vi "recipeScript getScriptInfo.vi"(0 "sysCode":string, 1 "method":T1) -> (3 "output":string)   [LabVIEW 2018]
uses:
  getScriptInfo.ctl
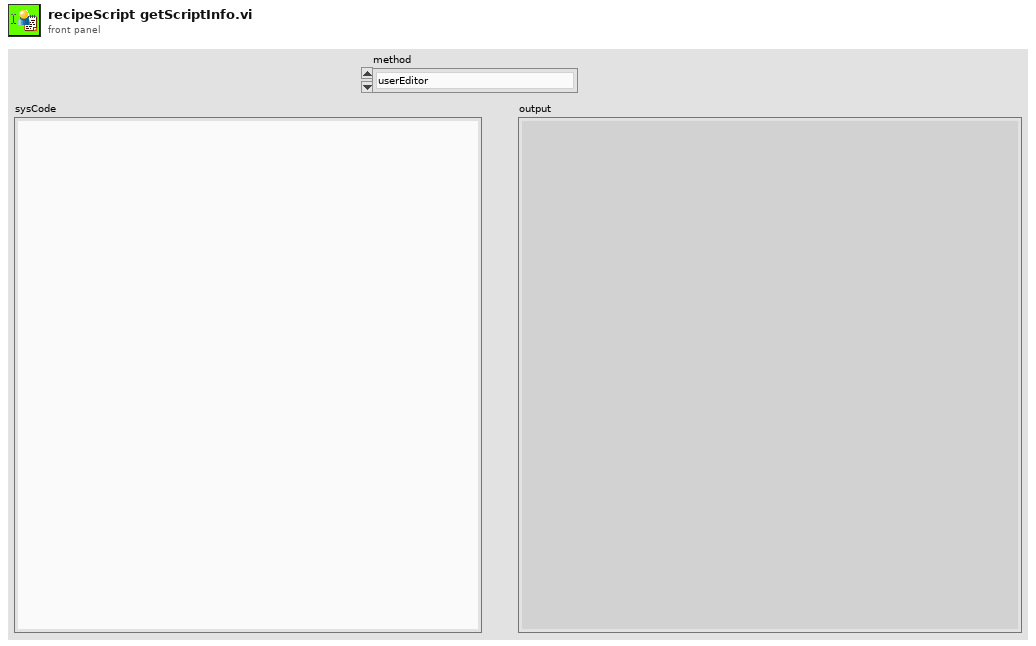
[diagram p1: front panel]
types:
  T1 = typedef "getScriptInfo.ctl" = enum16{"userEditor", "userParam", "instrParam", "sourcePath", "sourceTimeStamp", "versionInfo"}
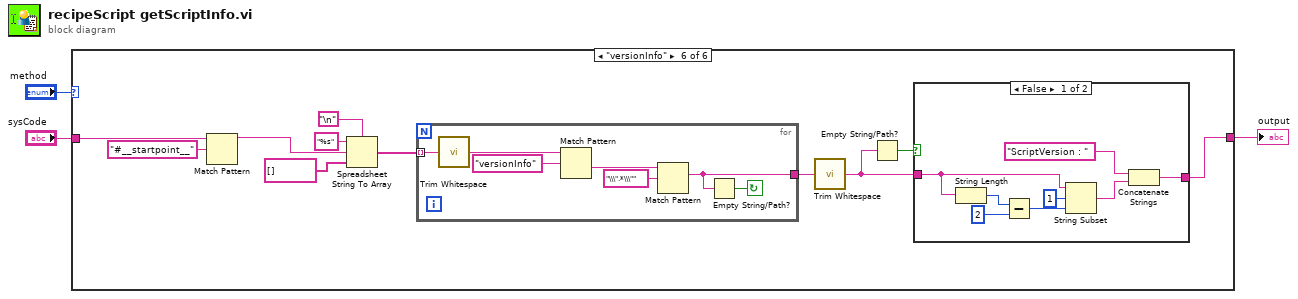
[diagram p0: block diagram]
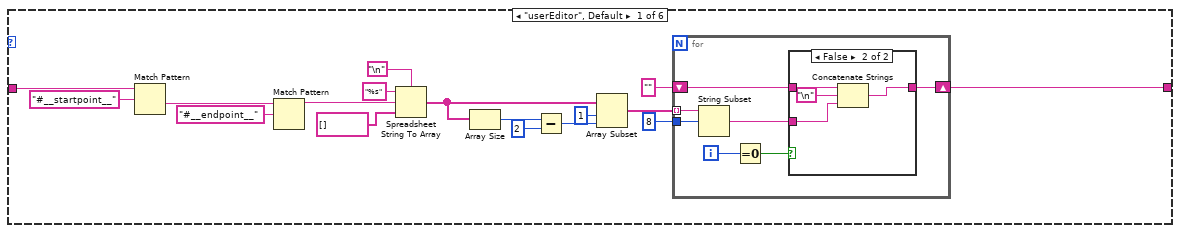
[diagram p2: hidden frame]
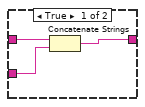
[diagram p3: hidden frame]
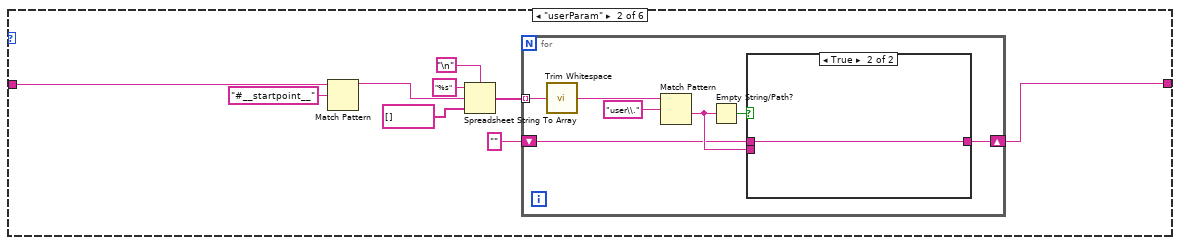
[diagram p4: hidden frame]
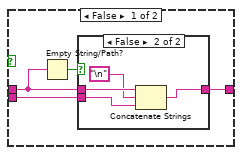
[diagram p5: hidden frame]
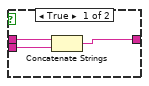
[diagram p6: hidden frame]
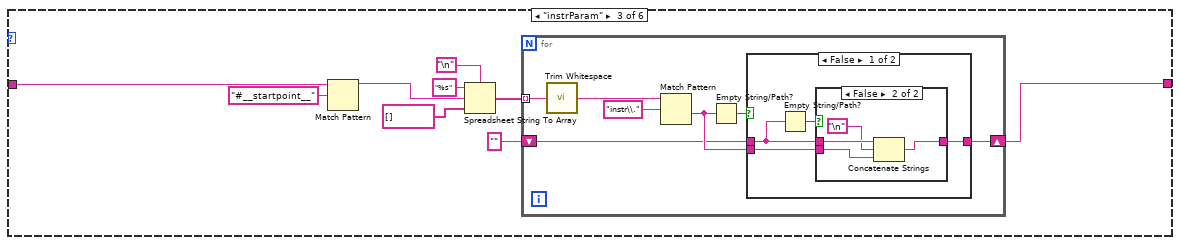
[diagram p7: hidden frame]
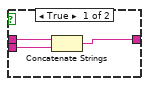
[diagram p8: hidden frame]
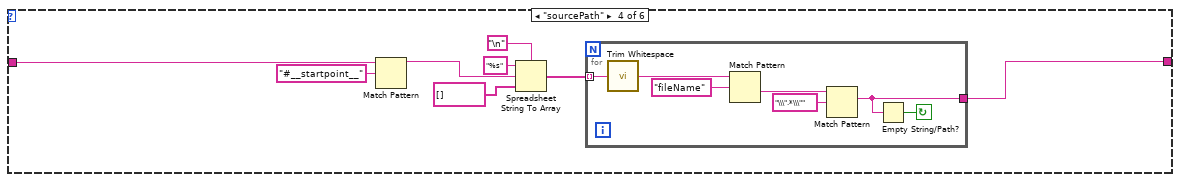
[diagram p10: hidden frame]
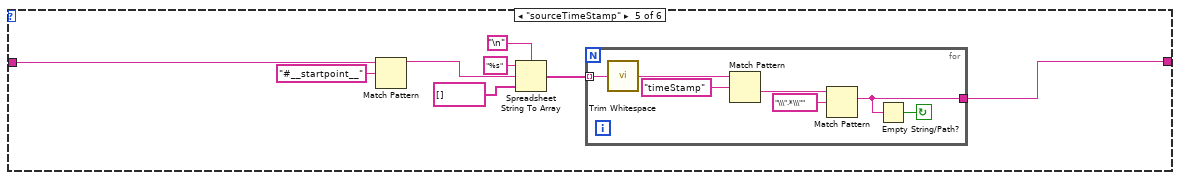
[diagram p11: hidden frame]
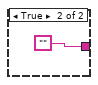
[diagram p12: hidden frame]
diagram:
  n1 = case shown="\"versionInfo\"" "method" {
    tunnel: "sysCode" -> [w20 w35 w63 w91 w106 w125]
    tunnel: [w8 w36 w64 w92 w107 w121] -> w2
    frame "userEditor", Default {
      n2 = Match Pattern(string=w20, regular expression="#__startpoint__") -> (after substring=w7:string)  [unwired: 1 in, 3 out]
      n3 = Match Pattern(string=w7, regular expression="#__endpoint__") -> (before substring=w5:string)  [unwired: 1 in, 3 out]
      n4 = Spreadsheet String To Array(delimiter (Tab)="\n", format string="%s", spreadsheet string=w5, array type (2D Dbl)=string[] []) -> (array=w14:string[])
      n5 = Array Size(array=w14) -> (size(s)=w13:i32)
      n6 = Subtract(x=w13, y=2) -> (x-y=w11:i32)
      n7 = Array Subset(array=w14, index=1, length=w11) -> (w10:string[])
      n8 = for {
        tunnel: w10 -> [w23] mode=indexing
        shift-right: [w26] -> w8
        shift-left: "" -> [w27]
        tunnel: 8 ("offset (0)") -> [w22]
        i -> [w25]
        n9 = String Subset(string=w23, offset (0)=w22) -> (substring=w21:string)  [unwired: 1 in]
        n10 = Equal To 0?(x=w25) -> (x = 0?=w24:bool)
        n11 = case shown="False" w24 {
          tunnel: w27 -> [w30 w34]
          tunnel: [w29 w33] -> w26
          tunnel: w21 -> [w28 w32]
          frame True {
            n12 = Concatenate Strings(w30, w28) -> (w29:string)
          }
          frame False {
            n13 = Concatenate Strings(w34, "\n", w32) -> (w33:string)
          }
        }
      }
    }
    frame "userParam" {
      n14 = Match Pattern(string=w35, regular expression="#__startpoint__") -> (before substring=w39:string)  [unwired: 1 in, 3 out]
      n15 = Spreadsheet String To Array(delimiter (Tab)="\n", format string="%s", spreadsheet string=w39, array type (2D Dbl)=string[] []) -> (array=w38:string[])
      n16 = for {
        tunnel: w38 -> [w50] mode=indexing
        shift-right: [w45] -> w36
        shift-left: "" -> [w44]
        n17 = call <vilib>:"Trim Whitespace.vi"("string"=w50) -> ("trimmed string"=w49:string)  [unwired: 1 in]
        n18 = Match Pattern(string=w49, regular expression="user\\.") -> (after substring=w46:string)  [unwired: 1 in, 3 out]
        n19 = Empty String/Path?(string/path=w46) -> (empty?=w47:bool)
        n20 = case shown="True" w47 {
          tunnel: w44 -> [w52 w62]
          tunnel: w46 -> [w54 _]
          tunnel: [w53 w62] -> w45
          frame False {
            n21 = Empty String/Path?(string/path=w52) -> (empty?=w51:bool)
            n22 = case shown="False" w51 {
              tunnel: w52 -> [w57 w61]
              tunnel: w54 -> [w56 w58]
              tunnel: [w55 w60] -> w53
              frame True {
                n23 = Concatenate Strings(w57, w56) -> (w55:string)
              }
              frame False {
                n24 = Concatenate Strings(w61, "\n", w58) -> (w60:string)
              }
            }
          }
          frame True {
          }
        }
      }
    }
    frame "instrParam" {
      n25 = Match Pattern(string=w63, regular expression="#__startpoint__") -> (before substring=w67:string)  [unwired: 1 in, 3 out]
      n26 = Spreadsheet String To Array(delimiter (Tab)="\n", format string="%s", spreadsheet string=w67, array type (2D Dbl)=string[] []) -> (array=w66:string[])
      n27 = for {
        tunnel: w66 -> [w78] mode=indexing
        shift-right: [w73] -> w64
        shift-left: "" -> [w72]
        n28 = call <vilib>:"Trim Whitespace.vi"("string"=w78) -> ("trimmed string"=w77:string)  [unwired: 1 in]
        n29 = Match Pattern(string=w77, regular expression="instr\\.") -> (after substring=w74:string)  [unwired: 1 in, 3 out]
        n30 = Empty String/Path?(string/path=w74) -> (empty?=w75:bool)
        n31 = case shown="False" w75 {
          tunnel: w72 -> [w80 w90]
          tunnel: w74 -> [w82 _]
          tunnel: [w81 w90] -> w73
          frame False {
            n32 = Empty String/Path?(string/path=w80) -> (empty?=w79:bool)
            n33 = case shown="False" w79 {
              tunnel: w80 -> [w85 w89]
              tunnel: w82 -> [w84 w86]
              tunnel: [w83 w88] -> w81
              frame True {
                n34 = Concatenate Strings(w85, w84) -> (w83:string)
              }
              frame False {
                n35 = Concatenate Strings(w89, "\n", w86) -> (w88:string)
              }
            }
          }
          frame True {
          }
        }
      }
    }
    frame "sourcePath" {
      n36 = Match Pattern(string=w91, regular expression="#__startpoint__") -> (before substring=w94:string)  [unwired: 1 in, 3 out]
      n37 = Spreadsheet String To Array(delimiter (Tab)="\n", format string="%s", spreadsheet string=w94, array type (2D Dbl)=string[] []) -> (array=w93:string[])
      n38 = for {
        tunnel: w93 -> [w103] mode=indexing
        tunnel: [w100] -> w92
        stop <- w99 continue-if-true
        n39 = call <vilib>:"Trim Whitespace.vi"("string"=w103) -> ("trimmed string"=w105:string)  [unwired: 1 in]
        n40 = Match Pattern(string=w105, regular expression="fileName") -> (after substring=w102:string)  [unwired: 1 in, 3 out]
        n41 = Match Pattern(string=w102, regular expression="\\\".*\\\"") -> (match substring=w100:string)  [unwired: 1 in, 3 out]
        n42 = Empty String/Path?(string/path=w100) -> (empty?=w99:bool)
      }
    }
    frame "sourceTimeStamp" {
      n43 = Match Pattern(string=w106, regular expression="#__startpoint__") -> (before substring=w109:string)  [unwired: 1 in, 3 out]
      n44 = Spreadsheet String To Array(delimiter (Tab)="\n", format string="%s", spreadsheet string=w109, array type (2D Dbl)=string[] []) -> (array=w108:string[])
      n45 = for {
        tunnel: w108 -> [w118] mode=indexing
        tunnel: [w115] -> w107
        stop <- w114 continue-if-true
        n46 = call <vilib>:"Trim Whitespace.vi"("string"=w118) -> ("trimmed string"=w120:string)  [unwired: 1 in]
        n47 = Match Pattern(string=w120, regular expression="timeStamp") -> (after substring=w117:string)  [unwired: 1 in, 3 out]
        n48 = Match Pattern(string=w117, regular expression="\\\".*\\\"") -> (match substring=w115:string)  [unwired: 1 in, 3 out]
        n49 = Empty String/Path?(string/path=w115) -> (empty?=w114:bool)
      }
    }
    frame "versionInfo" {
      n50 = Match Pattern(string=w125, regular expression="#__startpoint__") -> (before substring=w127:string)  [unwired: 1 in, 3 out]
      n51 = Spreadsheet String To Array(delimiter (Tab)="\n", format string="%s", spreadsheet string=w127, array type (2D Dbl)=string[] []) -> (array=w126:string[])
      n52 = for {
        tunnel: w126 -> [w145] mode=indexing
        tunnel: [w142] -> w122
        stop <- w141 continue-if-true
        n53 = call <vilib>:"Trim Whitespace.vi"("string"=w145) -> ("trimmed string"=w147:string)  [unwired: 1 in]
        n54 = Match Pattern(string=w147, regular expression="versionInfo") -> (after substring=w144:string)  [unwired: 1 in, 3 out]
        n55 = Match Pattern(string=w144, regular expression="\\\".*\\\"") -> (match substring=w142:string)  [unwired: 1 in, 3 out]
        n56 = Empty String/Path?(string/path=w142) -> (empty?=w141:bool)
      }
      n57 = call <vilib>:"Trim Whitespace.vi"("string"=w122) -> ("trimmed string"=w123:string)  [unwired: 1 in]
      n58 = Empty String/Path?(string/path=w123) -> (empty?=w124:bool)
      n59 = case shown="False" w124 {
        tunnel: [w132 ""] -> w121
        tunnel: w123 -> [w138 _]
        frame False {
          n60 = String Length(string=w138) -> (length=w137:i32)
          n61 = Subtract(x=w137, y=2) -> (x-y=w135:i32)
          n62 = String Subset(string=w138, offset (0)=1, length (rest)=w135) -> (substring=w133:string)
          n63 = Concatenate Strings("ScriptVersion : " ("regular expression"), w133) -> (w132:string)
        }
        frame True {
        }
      }
    }
  }
  "output" <- w2
